vi "Set Return Header.vi"(8 "error in (no error)":errorcluster, 9 "Value":string, 10 "Name":string, 11 "WebSockets in":refnum<class "WebSocket.lvclass">) -> (0 "error out":errorcluster, 3 "WebSockets out":refnum<class "WebSocket.lvclass">)   [LabVIEW 2013, in "WebSockets.lvlib" / "WebSocket.lvclass"]
doc: "Adds a single return header to the WebSocket object. Used internally to process the response headers."
uses:
  WebSocket.lvclass
  WebSocket.lvclass/WebSocket.ctl
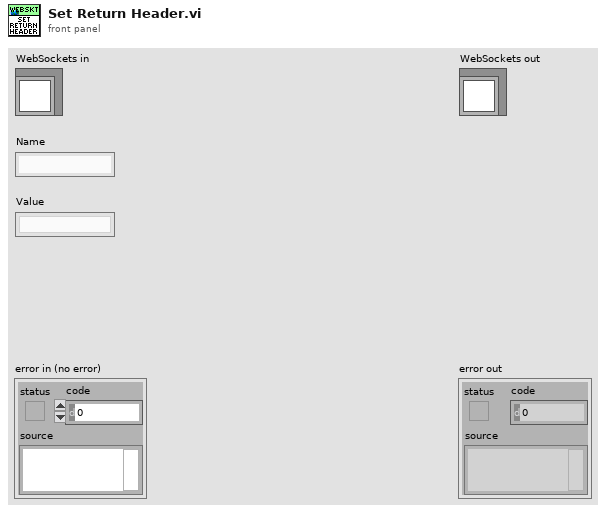
[diagram p1: front panel]
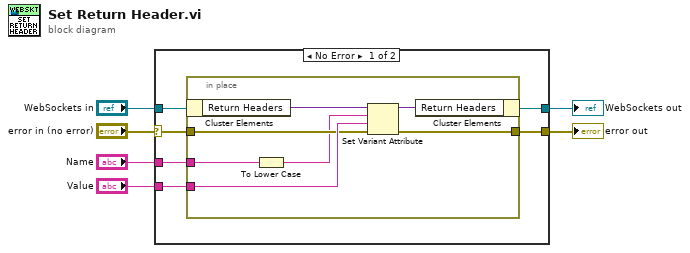
[diagram p0: block diagram]
diagram:
  n1 = case shown="No Error" "error in (no error)" {
    selector: "error in (no error)" -> [w8 w21]
    tunnel: [w7 w21] -> w5
    tunnel: [w11 w20] -> w3
    tunnel: "WebSockets in" -> [w12 w20]
    tunnel: "Name" -> [w10 _]
    tunnel: "Value" -> [w9 _]
    frame No Error {
      n2 = in-place {
        in-place-border: w10 -> [w17]
        in-place-border: w9 -> [w16]
        in-place-border: w8 -> [w15]
        in-place-border: [w14] -> w7
        n3 = in-place-cluster #1(w12) -> ("Return Headers"=w19:variant)
        n4 = To Lower Case(string=w17) -> (all lower case string=w13:string)
        n5 = Set Variant Attribute(Variant=w19, name=w13, value=w16, error in=w15) -> (Variant out=w18:variant, error out=w14:errorcluster)  [unwired: 1 out]
        n6 = in-place-cluster #1("Return Headers"=w18) -> (w11:refnum<class "WebSocket.lvclass">)
      }
    }
    frame Error {
    }
  }
  "error out" <- w5
  "WebSockets out" <- w3
